vi "WLAN Select and Initiate Measurements.vi"(0 "Instrument Handle In":refnum<k21>, 1 "Selector String":string, 2 "Result Name":string, 5 "Measurements":T2(array[ring]), 7 "Auto Level Configuration":T1={"Enabled"=FALSE, "Measurement Interval (s)"=0.01} {"Measurement Interval (s)" min=1e-06 max=100.0 format="%.2p"}, 11 "error in (no error)":errorcluster, 12 "Enable All Traces (F)":bool) -> (4 "Instrument Handle Out":refnum<k21>, 6 "Selector String Out":string, 15 "error out":errorcluster)   [LabVIEW 2016, in "RFmxWLAN.lvlib"]
uses:
  RFmxWLAN.lvlib
  Common/SA Auto Level Configuration.ctl
  <vilib>/RFmx/WLAN/mx/RFmxWLAN.llb/RFmxWLAN Select Measurement (Multiple).vi
  Common/Common.lvlib
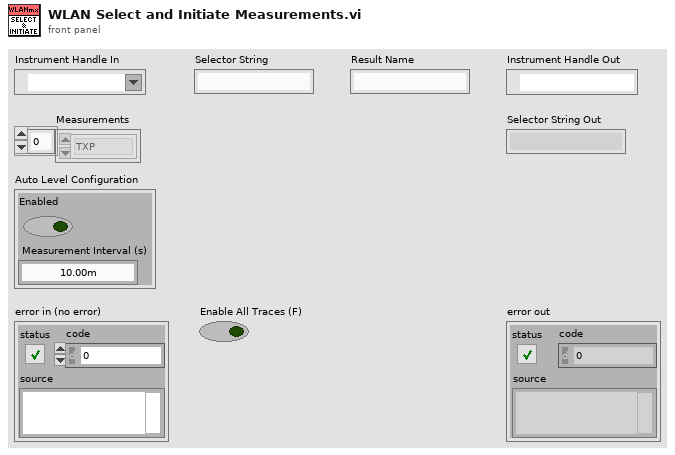
[diagram p1: front panel]
types:
  T1 = typedef "Common.lvlib/SA Auto Level Configuration.ctl" = cluster{"Enabled":bool, "Measurement Interval (s)":dbl}
  T2 = enum16{"TXP", "PowerRamp", "DSSSModAcc", "OFDMModAcc", "SEM"}[]
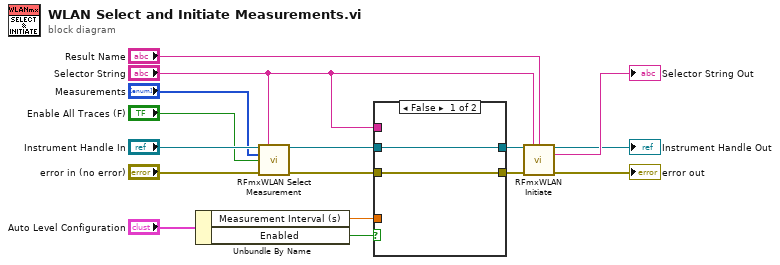
[diagram p0: block diagram]
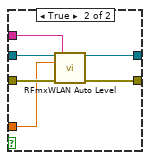
[diagram p2: hidden frame]
diagram:
  n1 = Unbundle By Name("Auto Level Configuration") -> ("Measurement Interval (s)"=w2:dbl, "Enabled"=w3:bool)
  n2 = call-poly <vilib>:"RFmxWLAN Select Measurement.vi"("Instrument Handle In"="Instrument Handle In", "Selector String"="Selector String", "Measurements"="Measurements", "Enable All Traces"="Enable All Traces (F)", "error in (no error)"="error in (no error)") -> ("Instrument Handle Out"=w6:refnum<k21>, "error out"=w13:errorcluster)  [unwired: 9 in]
  n3 = case shown="False" w3 {
    tunnel: w13 -> [w17 w24]
    tunnel: [w17 w23] -> w7
    tunnel: w6 -> [w18 w22]
    tunnel: [w18 w21] -> w5
    tunnel: w2 -> [_ w20]
    tunnel: "Selector String" -> [_ w19]
    frame False {
    }
    frame True {
      n4 = call <vilib>:"RFmxWLAN Auto Level.vi"("Instrument Handle In"=w22, "Selector String"=w19, "Measurement Interval (s)"=w20, "error in (no error)"=w24) -> ("Instrument Handle Out"=w21:refnum<k21>, "error out"=w23:errorcluster)  [unwired: 10 in]
    }
  }
  n5 = call <vilib>:"RFmxWLAN Initiate.vi"("Instrument Handle In"=w5, "Selector String"="Selector String", "Result Name"="Result Name", "error in (no error)"=w7) -> ("Instrument Handle Out"=→"Instrument Handle Out":refnum<k21>, "Selector String Out"=→"Selector String Out":string, "error out"=→"error out":errorcluster)  [unwired: 9 in]
